vi "Actor Core.vi"(8 "error in":errorcluster, 11 "Optimization Test in":refnum<class "Optimization Test.lvclass">) -> (0 "error out":errorcluster, 3 "Actor out":refnum<class "Actor.lvclass">)   [LabVIEW 2016, in "Optimization Framework Test.lvlib" / "Optimization Test.lvclass"]
doc: "(<B>Filename</B>: Actor Framework.lvlib:Actor.lvclass:Actor Core.vi)\n\nReceives messages to the actor, reacts to them, and initiates any error handling that may shut the actor down.\n\nDescendant classes may override this VI to append parallel tasks for the actor to complete while it handles messages. Overrides use the Call Parent Method node."
uses:
  Optimization Test.lvclass
  C:/Program Files (x86)/National Instruments/LabVIEW 2016/vi.lib/ActorFramework/Actor/Actor.lvclass
  <vilib>/ActorFramework/Actor/Actor.lvclass
  Optimization Framework/Optimization/Controls/Microgrid State Selector.ctl
  Optimization Framework/Optimization/Optimization.lvclass
  <vilib>/ActorFramework/Actor/Actor.lvclass/Actor.ctl
  <vilib>/ActorFramework/Message Enqueuer/Message Enqueuer.lvclass/Message Enqueuer.ctl
  Optimization Framework/Optimization Messages/Update Microgrid State Msg/Update Microgrid State Msg.lvclass/Update Microgrid State Msg.ctl
  Optimization Framework/Optimization/Controls/Optimization Parameters Line Configuration.ctl
  Optimization Framework/Optimization/Controls/Optimization Line Configuration Enum.ctl
  Optimization Framework/Optimization Messages/Update Device Line Configuration Msg/Update Device Line Configuration Msg.lvclass/Update Device Line Configuration Msg.ctl
  Optimization Framework/Optimization/Controls/Measurement Cluster Energy Storage.ctl
  Optimization Framework/Optimization/Controls/3-phase Cluster.ctl
  Optimization Framework/Optimization Messages/Update Energy Storage Measurement Msg/Update Energy Storage Measurement Msg.lvclass/Update Energy Storage Measurement Msg.ctl
  Optimization Framework/Optimization/Controls/Optimization Parameters Energy Storage.ctl
  Optimization Framework/Optimization/Controls/Device Control Capabilities.ctl
  Optimization Framework/Optimization Messages/Update Energy Storage Parameter Msg/Update Energy Storage Parameter Msg.lvclass/Update Energy Storage Parameter Msg.ctl
  Optimization Framework/Optimization/Controls/Measurement Cluster Generator.ctl
  Optimization Framework/Optimization Messages/Update Generator Measurement Msg/Update Generator Measurement Msg.lvclass/Update Generator Measurement Msg.ctl
  Optimization Framework/Optimization/Controls/Optimization Parameters Generator.ctl
  Master Controller Core/Master Controller/Controls/Current Status.ctl
  Optimization Framework/Optimization Messages/Update Generator Parameter Msg/Update Generator Parameter Msg.lvclass/Update Generator Parameter Msg.ctl
  Optimization Framework/Optimization/Controls/Forecast Device Power.ctl
  Optimization Framework/Optimization/Controls/PDF Cluster.ctl
  Optimization Framework/Optimization Messages/Update Load Forecast Longterm Msg/Update Load Forecast Longterm Msg.lvclass/Update Load Forecast Longterm Msg.ctl
  Optimization Framework/Optimization Messages/Update Load Forecast Shortterm Msg/Update Load Forecast Shortterm Msg.lvclass/Update Load Forecast Shortterm Msg.ctl
  Optimization Framework/Optimization Messages/Update PCC DeviceID Msg/Update PCC DeviceID Msg.lvclass/Update PCC DeviceID Msg.ctl
  Optimization Framework/Optimization/Controls/Schedule Price.ctl
  Optimization Framework/Optimization Messages/Update Price Schedule Msg/Update Price Schedule Msg.lvclass/Update Price Schedule Msg.ctl
  Optimization Framework/Optimization Messages/Update PV Forecast Longterm Msg/Update PV Forecast Longterm Msg.lvclass/Update PV Forecast Longterm Msg.ctl
  Optimization Framework/Optimization Messages/Update PV Forecast Shortterm Msg/Update PV Forecast Shortterm Msg.lvclass/Update PV Forecast Shortterm Msg.ctl
  Optimization Framework/Optimization/Controls/Measurement Cluster PV.ctl
  Optimization Framework/Optimization Messages/Update PV Measurement Msg/Update PV Measurement Msg.lvclass/Update PV Measurement Msg.ctl
  Optimization Framework/Optimization/Controls/Measurement Cluster Smart Relay.ctl
  Optimization Framework/Optimization Messages/Update Smart Relay Measurement Msg/Update Smart Relay Measurement Msg.lvclass/Update Smart Relay Measurement Msg.ctl
  <vilib>/ActorFramework/Message Enqueuer/Init from Existing Queue.vi
  <vilib>/ActorFramework/Message Enqueuer/Enqueue.vi
  Optimization Framework/Optimization Messages/Update Microgrid State Msg/Update Microgrid State Msg.lvclass
  C:/Program Files (x86)/National Instruments/LabVIEW 2016/vi.lib/ActorFramework/Message/Message.lvclass
  Optimization Framework/Optimization Messages/Update Device Line Configuration Msg/Update Device Line Configuration Msg.lvclass
  Optimization Framework/Optimization Messages/Update Energy Storage Measurement Msg/Update Energy Storage Measurement Msg.lvclass
  Optimization Framework/Optimization Messages/Update Energy Storage Parameter Msg/Update Energy Storage Parameter Msg.lvclass
  Optimization Framework/Optimization Messages/Update Generator Measurement Msg/Update Generator Measurement Msg.lvclass
  Optimization Framework/Optimization Messages/Update Generator Parameter Msg/Update Generator Parameter Msg.lvclass
  Optimization Framework/Optimization Messages/Update Load Forecast Longterm Msg/Update Load Forecast Longterm Msg.lvclass
  Optimization Framework/Optimization Messages/Update Load Forecast Shortterm Msg/Update Load Forecast Shortterm Msg.lvclass
  Optimization Framework/Optimization Messages/Update PCC DeviceID Msg/Update PCC DeviceID Msg.lvclass
  Optimization Framework/Optimization Messages/Update Price Schedule Msg/Update Price Schedule Msg.lvclass
  Optimization Framework/Optimization Messages/Update PV Forecast Longterm Msg/Update PV Forecast Longterm Msg.lvclass
  Optimization Framework/Optimization Messages/Update PV Forecast Shortterm Msg/Update PV Forecast Shortterm Msg.lvclass
  Optimization Framework/Optimization Messages/Update PV Measurement Msg/Update PV Measurement Msg.lvclass
  Optimization Framework/Optimization Messages/Update Smart Relay Measurement Msg/Update Smart Relay Measurement Msg.lvclass
  <vilib>/ActorFramework/Stop Msg/Stop Msg.lvclass
  <vilib>/ActorFramework/Message Priority Queue/Priority Enqueue.vi
  <vilib>/ActorFramework/Message Enqueuer/Message Enqueuer.lvclass
  Master Controller Core/Master Controller/Master Controller.lvclass
panel:
  in  "Data Type":T1(ring)
  in  "Send Data":bool
  in  "Microgrid State":T2
  in  "Execute":bool
  in  "Stop Button":bool
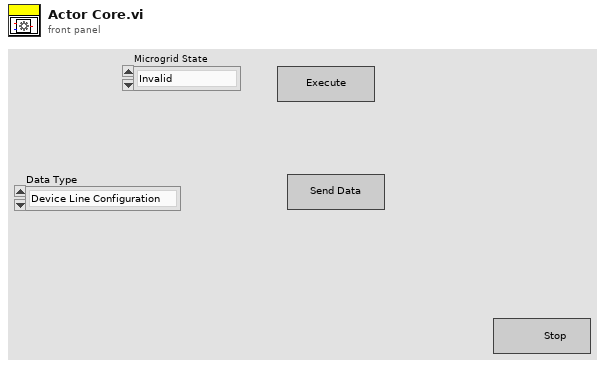
[diagram p1: front panel]
types:
  T1 = enum16{"Device Line Configuration", "ES Measurements", "ES Parameters", "Generator Measurements", "Generator Parameters", "Load Forecast Longterm", "Load Forecast Shortterm", "PCC DeviceID", "Price Schedule", "PV Forecast Longterm", "PV Forecast Shortterm", "PV Measurement", "Smart Relay Measurement"}
  T2 = typedef "Optimization Framework.lvlib/Optimization.lvclass/Microgrid State Selector.ctl" = enum16{"Invalid", "Commissioning", "Activation", "Blackstart", "OnGrid", "OffGrid", "Islanding", "Resynchronization", "Shutdown"}
  T3 = typedef "Optimization Framework.lvlib/Optimization.lvclass/Optimization Parameters Line Configuration.ctl" = cluster{"DeviceID":u64, "Line Configuration":T4}
  T4 = typedef "Optimization Framework.lvlib/Optimization.lvclass/Optimization Line Configuration Enum.ctl" = enum8{"Invalid", "L-L", "L-N", "L-G"}
  T5 = typedef "Optimization Framework.lvlib/Optimization.lvclass/Measurement Cluster Energy Storage.ctl" = cluster{"Device ID":u64, "SOC":dbl, "Voltage":T6, "Current":T6, "Real Power":T6, "Reactive Power":T6}
  T6 = typedef "Optimization Framework.lvlib/Optimization.lvclass/3-phase Cluster.ctl" = cluster{"Phase A":dbl, "Phase B":dbl, "Phase C":dbl}
  T7 = typedef "Optimization Framework.lvlib/Optimization.lvclass/Optimization Parameters Energy Storage.ctl" = cluster{"Device ID":u64, "Bus ID":u16, "Voltage (V)":dbl, "Power Rating (kVA)":dbl, "Energy Rating (kWh)":dbl, "Ramp Rate (kW/s)":dbl, "Max Power Factor (leading)":dbl, "Max Power Factor (lagging)":dbl, "Charging Efficiency Curve Power":dbl[], "Charging Efficiency Curve Efficiency":dbl[], "Discharging Efficiency Curve Power":dbl[], "Discharging Efficiency Curve Efficiency":dbl[], "Min SOC(%)":dbl, "Max SOC(%)":dbl, "Start SOC(%)":dbl, "End SOC(%)":dbl, "Control Capabilities":T8}
  T8 = typedef "Optimization Framework.lvlib/Optimization.lvclass/Device Control Capabilities.ctl" = cluster{"VF":bool, "P":bool, "Q":bool, "PF":bool, "PV":bool}
  T9 = typedef "Optimization Framework.lvlib/Optimization.lvclass/Measurement Cluster Generator.ctl" = cluster{"Device ID":u64, "Voltage":T6, "Current":T6, "Real Power":T6, "Reactive Power":T6}
  T10 = typedef "Optimization Framework.lvlib/Optimization.lvclass/Optimization Parameters Generator.ctl" = cluster{"Device ID ":u64, "Bus ID":u16, "Voltage (V)":dbl, "Min Power (kVA)":dbl, "Power Rating (kVA)":dbl, "Ramp Rate (kW/s)":dbl, "Max PF Magnitude (leading)":dbl, "Max PF Magnitude (lagging)":dbl, "Efficiency Curve Power":dbl[], "Efficiency Curve Efficiency":dbl[], "Start-up Time (s)":dbl, "Start-up Cost":dbl, "Fuel Cost":dbl, "Current Status":T11, "Control Capabilities":T8}
  T11 = typedef "Master Controller Core.lvlib/Master Controller.lvclass/Current Status.ctl" = enum8{"Off", "On"}
  T12 = typedef "Optimization Framework.lvlib/Optimization.lvclass/Forecast Device Power.ctl" = cluster{"Device ID":u64, "t0":timestamp, "dt":dbl, "Power Array":dbl[], "Minimum Power Array":dbl[], "Maximum Power Array":dbl[], "PDF Array":T13[]}
  T13 = typedef "Optimization Framework.lvlib/Optimization.lvclass/PDF Cluster.ctl" = cluster{"P0":dbl, "dP":dbl, "Probability Array":dbl[]}
  T14 = typedef "Optimization Framework.lvlib/Optimization.lvclass/Schedule Price.ctl" = cluster{"t0":timestamp, "dt":dbl, "Price Array":dbl[], "Demand Charge":dbl, "Demand Charge Duration":dbl}
  T15 = typedef "Optimization Framework.lvlib/Optimization.lvclass/Measurement Cluster PV.ctl" = cluster{"Device ID":u64, "Irradiance":dbl, "Voltage":T6, "Current":T6, "Real Power":T6, "Reactive Power":T6}
  T16 = typedef "Optimization Framework.lvlib/Optimization.lvclass/Measurement Cluster Smart Relay.ctl" = cluster{"Device ID":u64, "Voltage":T6, "Voltage 2":T6, "Current":T6, "Real Power":T6, "Reactive Power":T6}
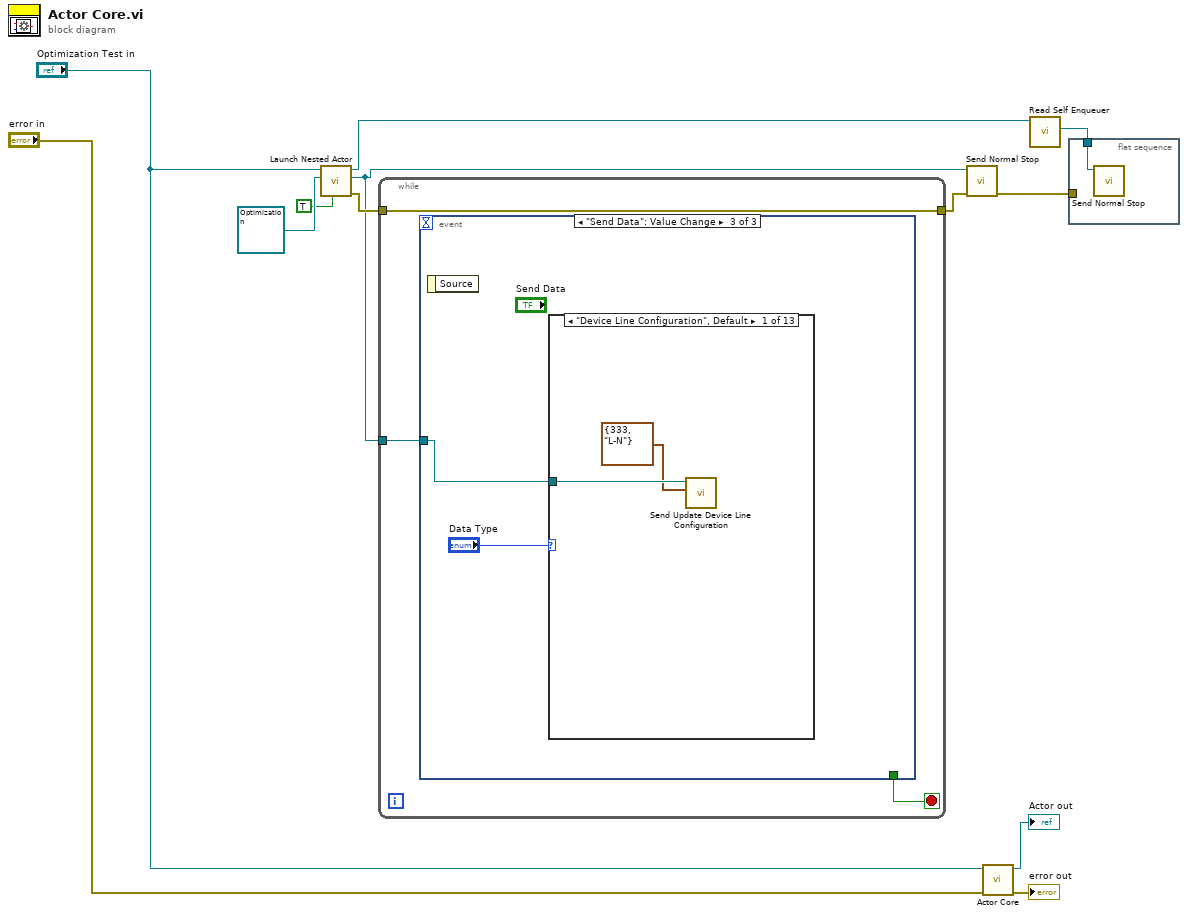
[diagram p0: block diagram]
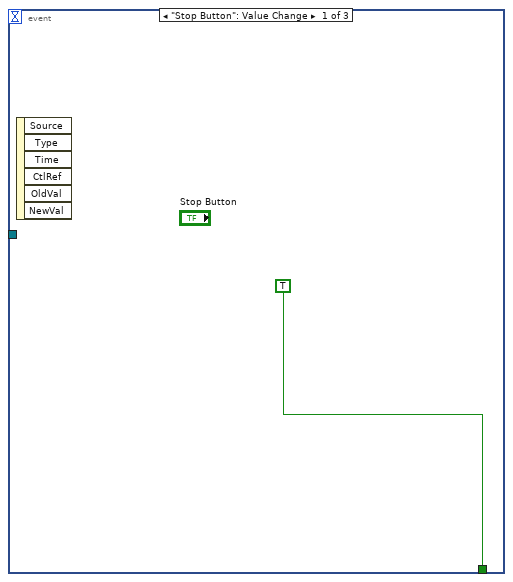
[diagram p2: hidden frame]
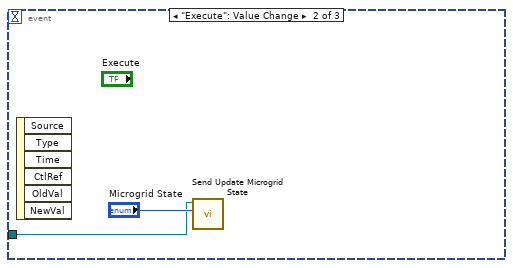
[diagram p3: hidden frame]
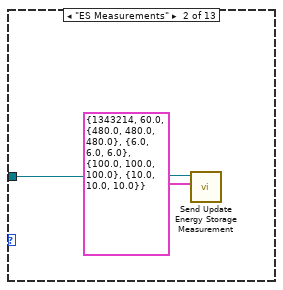
[diagram p4: hidden frame]
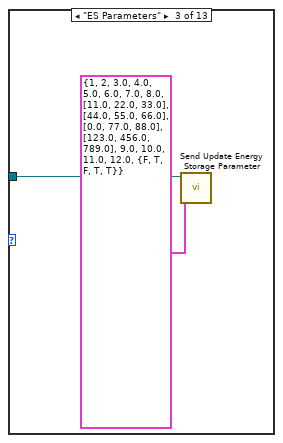
[diagram p5: hidden frame]
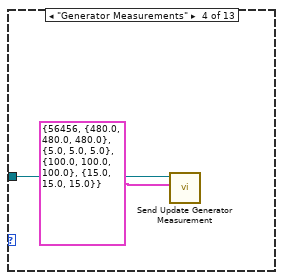
[diagram p6: hidden frame]
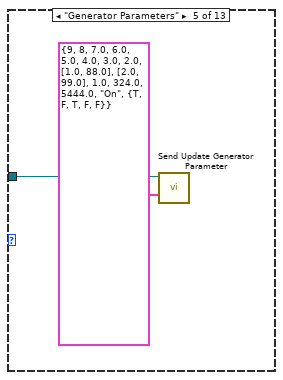
[diagram p7: hidden frame]
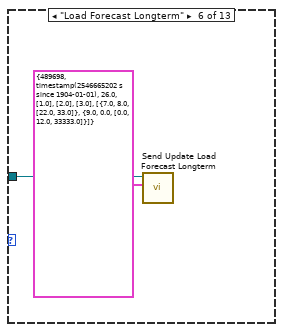
[diagram p8: hidden frame]
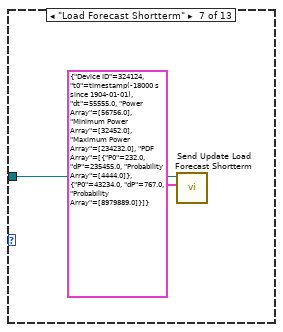
[diagram p9: hidden frame]
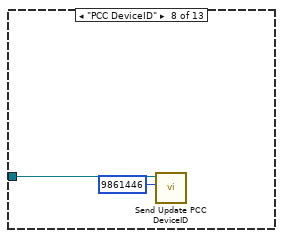
[diagram p10: hidden frame]
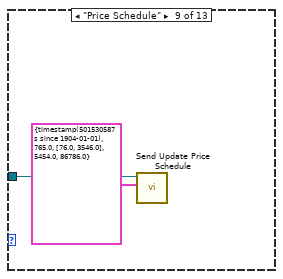
[diagram p11: hidden frame]
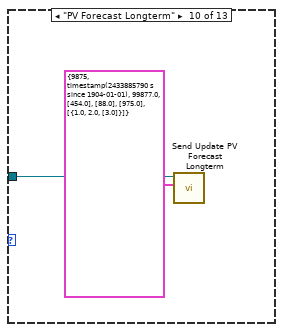
[diagram p12: hidden frame]
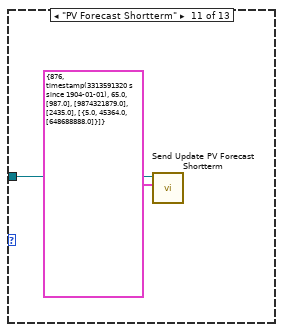
[diagram p13: hidden frame]
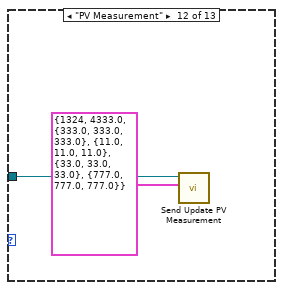
[diagram p14: hidden frame]
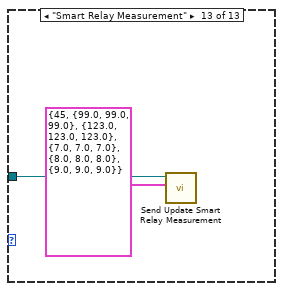
[diagram p15: hidden frame]
diagram:
  n1 = call <vilib>:"Launch Nested Actor.vi"("Open Actor Core front panel? (F)"=TRUE, "Nested Actor"=refnum<class "Optimization.lvclass"> refnum ("Optimization Framework.lvlib:Optimization.lvclass"), "Caller Actor in"="Optimization Test in") -> ("error out"=w3:errorcluster, "Nested Actor's Enqueuer"=w1:refnum<class "Message Enqueuer.lvclass">, "Caller Actor out"=w6:refnum<class "Optimization Test.lvclass">)  [unwired: 6 in]
  n2 = while {
    tunnel: w3 -> [w14]
    tunnel: [w14] -> w2
    tunnel: w1 -> [w13]
    stop <- w15 stop-if-true
    n3 = event shown="[2] \"Send Data\": Value Change" {
      selector: _ -> [_ _ _]
      dyn-events: _ -> [_ _ _]
      timeout: _ -> [_ _ _]
      tunnel: [TRUE _ _] -> w15
      tunnel: w13 -> [_ w17 w20]
      event "Stop Button": Value Change {
        n4 = event-data() -> ()  [unwired: 1 in, 6 out]
      }
      event "Execute": Value Change {
        n5 = event-data() -> ()  [unwired: 1 in, 6 out]
        n6 = call "Send Update Microgrid State.vi"("Microgrid State"="Microgrid State", "Message Enqueuer"=w17) -> ()  [unwired: 8 in, 2 out]
      }
      event "Send Data": Value Change {
        n7 = event-data() -> ()  [unwired: 1 in, 1 out]
        n8 = case shown="\"Device Line Configuration\", Default" "Data Type" {
          tunnel: w20 -> [w22 w24 w26 w28 w30 w32 w34 w36 w38 w40 w42 w44 w46]
          frame "Device Line Configuration", Default {
            n9 = call "Send Update Device Line Configuration.vi"("Line Configuration"=T3 {"DeviceID"=333, "Line Configuration"=enum."L-N"}, "Message Enqueuer"=w22) -> ()  [unwired: 8 in, 2 out]
          }
          frame "ES Measurements" {
            n10 = call "Send Update Energy Storage Measurement.vi"("Energy Storage Measurement"=T5 {"Device ID"=1343214, "SOC"=60.0, "Voltage"={"Phase A"=480.0, "Phase B"=480.0, "Phase C"=480.0}, "Current"={"Phase A"=6.0, "Phase B"=6.0, "Phase C"=6.0}, "Real Power"={"Phase A"=100.0, "Phase B"=100.0, "Phase C"=100.0}, "Reactive Power"={"Phase A"=10.0, "Phase B"=10.0, "Phase C"=10.0}}, "Message Enqueuer"=w24) -> ()  [unwired: 8 in, 2 out]
          }
          frame "ES Parameters" {
            n11 = call "Send Update Energy Storage Parameter.vi"("Energy Storage Parameters"=T7 {"Device ID"=1, "Bus ID"=2, "Voltage (V)"=3.0, "Power Rating (kVA)"=4.0, "Energy Rating (kWh)"=5.0, "Ramp Rate (kW/s)"=6.0, "Max Power Factor (leading)"=7.0, "Max Power Factor (lagging)"=8.0, "Charging Efficiency Curve Power"=[11.0, 22.0, 33.0], "Charging Efficiency Curve Efficiency"=[44.0, 55.0, 66.0], "Discharging Efficiency Curve Power"=[0.0, 77.0, 88.0], "Discharging Efficiency Curve Efficiency"=[123.0, 456.0, 789.0], "Min SOC(%)"=9.0, "Max SOC(%)"=10.0, "Start SOC(%)"=11.0, "End SOC(%)"=12.0, "Control Capabilities"={"VF"=FALSE, "P"=TRUE, "Q"=FALSE, "PF"=TRUE, "PV"=TRUE}}, "Message Enqueuer"=w26) -> ()  [unwired: 8 in, 2 out]
          }
          frame "Generator Measurements" {
            n12 = call "Send Update Generator Measurement.vi"("Generator Measurement"=T9 {"Device ID"=56456, "Voltage"={"Phase A"=480.0, "Phase B"=480.0, "Phase C"=480.0}, "Current"={"Phase A"=5.0, "Phase B"=5.0, "Phase C"=5.0}, "Real Power"={"Phase A"=100.0, "Phase B"=100.0, "Phase C"=100.0}, "Reactive Power"={"Phase A"=15.0, "Phase B"=15.0, "Phase C"=15.0}}, "Message Enqueuer"=w28) -> ()  [unwired: 8 in, 2 out]
          }
          frame "Generator Parameters" {
            n13 = call "Send Update Generator Parameter.vi"("Generator Parameters"=T10 {"Device ID "=9, "Bus ID"=8, "Voltage (V)"=7.0, "Min Power (kVA)"=6.0, "Power Rating (kVA)"=5.0, "Ramp Rate (kW/s)"=4.0, "Max PF Magnitude (leading)"=3.0, "Max PF Magnitude (lagging)"=2.0, "Efficiency Curve Power"=[1.0, 88.0], "Efficiency Curve Efficiency"=[2.0, 99.0], "Start-up Time (s)"=1.0, "Start-up Cost"=324.0, "Fuel Cost"=5444.0, "Current Status"=enum."On", "Control Capabilities"={"VF"=TRUE, "P"=FALSE, "Q"=TRUE, "PF"=FALSE, "PV"=FALSE}}, "Message Enqueuer"=w30) -> ()  [unwired: 8 in, 2 out]
          }
          frame "Load Forecast Longterm" {
            n14 = call "Send Update Load Forecast Longterm.vi"("Load Power Forecast"=T12 {"Device ID"=489698, "t0"=timestamp(2546665202 s since 1904-01-01), "dt"=26.0, "Power Array"=[1.0], "Minimum Power Array"=[2.0], "Maximum Power Array"=[3.0], "PDF Array"=[{"P0"=7.0, "dP"=8.0, "Probability Array"=[22.0, 33.0]}, {"P0"=9.0, "dP"=0.0, "Probability Array"=[0.0, 12.0, 33333.0]}]}, "Message Enqueuer"=w32) -> ()  [unwired: 8 in, 2 out]
          }
          frame "Load Forecast Shortterm" {
            n15 = call "Send Update Load Forecast Shortterm.vi"("Load Power Forecast"=T12 {"Device ID"=324124, "t0"=timestamp(-18000 s since 1904-01-01), "dt"=55555.0, "Power Array"=[56756.0], "Minimum Power Array"=[32452.0], "Maximum Power Array"=[234232.0], "PDF Array"=[{"P0"=232.0, "dP"=235455.0, "Probability Array"=[4444.0]}, {"P0"=43234.0, "dP"=767.0, "Probability Array"=[8979889.0]}]}, "Message Enqueuer"=w34) -> ()  [unwired: 8 in, 2 out]
          }
          frame "PCC DeviceID" {
            n16 = call "Send Update PCC DeviceID.vi"("PCC DeviceID"=u64 9861446, "Message Enqueuer"=w36) -> ()  [unwired: 8 in, 2 out]
          }
          frame "Price Schedule" {
            n17 = call "Send Update Price Schedule.vi"("Price Schedule"=T14 {"t0"=timestamp(501530587 s since 1904-01-01), "dt"=765.0, "Price Array"=[76.0, 3546.0], "Demand Charge"=5454.0, "Demand Charge Duration"=86786.0}, "Message Enqueuer"=w38) -> ()  [unwired: 8 in, 2 out]
          }
          frame "PV Forecast Longterm" {
            n18 = call "Send Update PV Forecast Longterm.vi"("Device Power Forecast"=T12 {"Device ID"=9875, "t0"=timestamp(2433885790 s since 1904-01-01), "dt"=99877.0, "Power Array"=[454.0], "Minimum Power Array"=[88.0], "Maximum Power Array"=[975.0], "PDF Array"=[{"P0"=1.0, "dP"=2.0, "Probability Array"=[3.0]}]}, "Message Enqueuer"=w40) -> ()  [unwired: 8 in, 2 out]
          }
          frame "PV Forecast Shortterm" {
            n19 = call "Send Update PV Forecast Shortterm.vi"("PV Power Forecast"=T12 {"Device ID"=876, "t0"=timestamp(3313591320 s since 1904-01-01), "dt"=65.0, "Power Array"=[987.0], "Minimum Power Array"=[9874321879.0], "Maximum Power Array"=[2435.0], "PDF Array"=[{"P0"=5.0, "dP"=45364.0, "Probability Array"=[648688888.0]}]}, "Message Enqueuer"=w42) -> ()  [unwired: 8 in, 2 out]
          }
          frame "PV Measurement" {
            n20 = call "Send Update PV Measurement.vi"("PV Forecast"=T15 {"Device ID"=1324, "Irradiance"=4333.0, "Voltage"={"Phase A"=333.0, "Phase B"=333.0, "Phase C"=333.0}, "Current"={"Phase A"=11.0, "Phase B"=11.0, "Phase C"=11.0}, "Real Power"={"Phase A"=33.0, "Phase B"=33.0, "Phase C"=33.0}, "Reactive Power"={"Phase A"=777.0, "Phase B"=777.0, "Phase C"=777.0}}, "Message Enqueuer"=w44) -> ()  [unwired: 8 in, 2 out]
          }
          frame "Smart Relay Measurement" {
            n21 = call "Send Update Smart Relay Measurement.vi"("Relay Measurement"=T16 {"Device ID"=45, "Voltage"={"Phase A"=99.0, "Phase B"=99.0, "Phase C"=99.0}, "Voltage 2"={"Phase A"=123.0, "Phase B"=123.0, "Phase C"=123.0}, "Current"={"Phase A"=7.0, "Phase B"=7.0, "Phase C"=7.0}, "Real Power"={"Phase A"=8.0, "Phase B"=8.0, "Phase C"=8.0}, "Reactive Power"={"Phase A"=9.0, "Phase B"=9.0, "Phase C"=9.0}}, "Message Enqueuer"=w46) -> ()  [unwired: 8 in, 2 out]
          }
        }
      }
    }
  }
  n22 = call <vilib>:"Send Normal Stop.vi"("error in (no error)"=w2, "Message Enqueuer"=w1) -> ("error out"=w4:errorcluster)  [unwired: 9 in]
  n23 = call-parent "Actor Core.vi"("error in"="error in", "Actor in"="Optimization Test in") -> ("error out"=→"error out":errorcluster, "Actor out"=→"Actor out":refnum<class "Actor.lvclass">)  [unwired: 8 in]
  n24 = call <vilib>:"Read Self Enqueuer.vi"("Actor"=w6) -> ("Self Enqueuer"=w5:refnum<class "Message Enqueuer.lvclass">)  [unwired: 10 in]
  n25 = flat-sequence {
    tunnel: w5 -> [w47]
    tunnel: w4 -> [_]
    frame #0 {
      n26 = call <vilib>:"Send Normal Stop.vi"("Message Enqueuer"=w47) -> ()  [unwired: 10 in, 1 out]
    }
  }
